vi "Configure Custom Real Time Noise.vi"(5 "Enable Real-Time AWGN (F: Disable)":bool, 6 "Noise Control Mode (0: Carrier+Noise)":i32(ring) items=["Carrier+Noise", "Carrier", "Noise"], 7 "Carrier/Noise Ratio (0 dB)":dbl, 8 "error in (no error)":errorcluster, 9 "Carrier Bandwidth (1 Hz)":dbl=1.0, 10 "Noise Bandwidth (1 Hz)":dbl=1.0, 11 "VISA resource name":refnum<visa-resource-name>) -> (0 "error out":errorcluster, 3 "VISA resource name out":refnum<visa-resource-name>)   [LabVIEW 2014, in "Agilent PSG MXG Series.lvlib"]
doc: "Configure real time noise settings.\n\n<B>Notes:</B>\n(1) This VI is valid only in N5172B and N5182B that install <B>Option 431</B> or <B>Option 403</B>."
uses:
  Agilent PSG MXG Series.lvlib
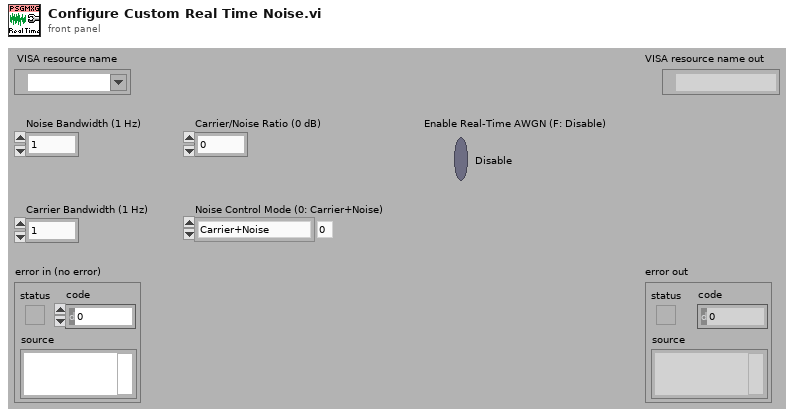
[diagram p1: front panel]
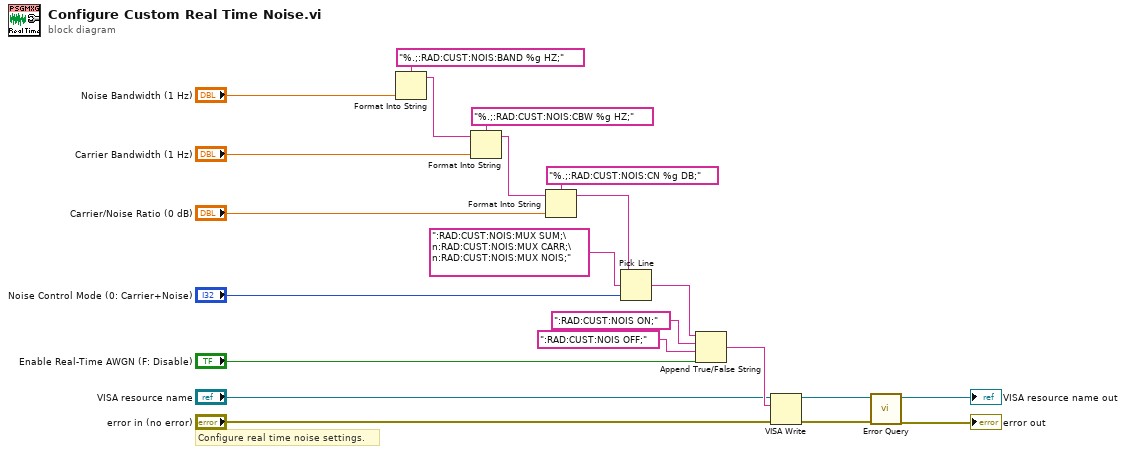
[diagram p0: block diagram]
diagram:
  # "Configure real time noise settings."
  n1 = Format Into String(format string="%.;:RAD:CUST:NOIS:BAND %g HZ;", "Noise Bandwidth (1 Hz)") -> (resulting string=w20:string)  [unwired: 2 in, 1 out]
  n2 = Format Into String(format string="%.;:RAD:CUST:NOIS:CBW %g HZ;", initial string=w20, "Carrier Bandwidth (1 Hz)") -> (resulting string=w17:string)  [unwired: 1 in, 1 out]
  n3 = Format Into String(format string="%.;:RAD:CUST:NOIS:CN %g DB;", initial string=w17, "Carrier/Noise Ratio (0 dB)") -> (resulting string=w12:string)  [unwired: 1 in, 1 out]
  n4 = Pick Line(string ("")=w12, multi-line string=":RAD:CUST:NOIS:MUX SUM;\n:RAD:CUST:NOIS:MUX CARR;\n:RAD:CUST:NOIS:MUX NOIS;", line index="Noise Control Mode (0: Carrier+Noise)") -> (output string=w11:string)
  n5 = Append True/False String(1:"Enable Real-Time AWGN (F: Disable)", 2:":RAD:CUST:NOIS OFF;", 3:":RAD:CUST:NOIS ON;", 4:w11) -> (0:w7:string)
  n6 = VISA Write(VISA resource name="VISA resource name", write buffer=w7, error in (no error)="error in (no error)") -> (VISA resource name out=w4:refnum<visa-resource-name>, error out=w3:errorcluster)  [unwired: 1 out]
  n7 = call "Error Query.vi"("error in (no error)"=w3, "VISA resource name"=w4) -> ("error out"=→"error out":errorcluster, "VISA resource name out"=→"VISA resource name out":refnum<visa-resource-name>)  [unwired: 8 out]
